vi "ODMR (with vol values).vi"() -> ()   [LabVIEW 2025]
uses:
  <vilib>/DAQmx/write.llb/DAQmx Write (Analog DBL 1Chan 1Samp).vi
  <vilib>/DAQmx/read.llb/DAQmx Read (Counter DBL 1Chan 1Samp).vi
  <vilib>/DAQmx/write.llb/DAQmx Write (Analog 1D DBL NChan 1Samp).vi
  <vilib>/DAQmx/create/channels.llb/DAQmx Create Channel (CI-Count Edges).vi
  <vilib>/DAQmx/create/channels.llb/DAQmx Create Channel (AO-Voltage-Basic).vi
  <vilib>/DAQmx/miscellaneous.llb/DAQmx Fill In Error Info.vi
  <vilib>/Utility/file.llb/Write Delimited Spreadsheet (DBL).vi
panel:
  in  "file path (dialog if empty)":path
  in  "MW stabalisation (ms)":u32
  out "interations":i32
  in  "Vx":dbl
  in  "Vy":dbl
  in  "End frequency (Ghz)":dbl
  in  "start frequency (Ghz)":dbl
  in  "Step size (Mhz)":dbl
  in  "Dwell time (ms)":u32=30
  out "XY Graph":cluster{"Y":dbl[], "Y":dbl[]}[](graph)
  out "appended array":dbl[](array[numeric])
  in  "VISA resource name":refnum<visa-resource-name>
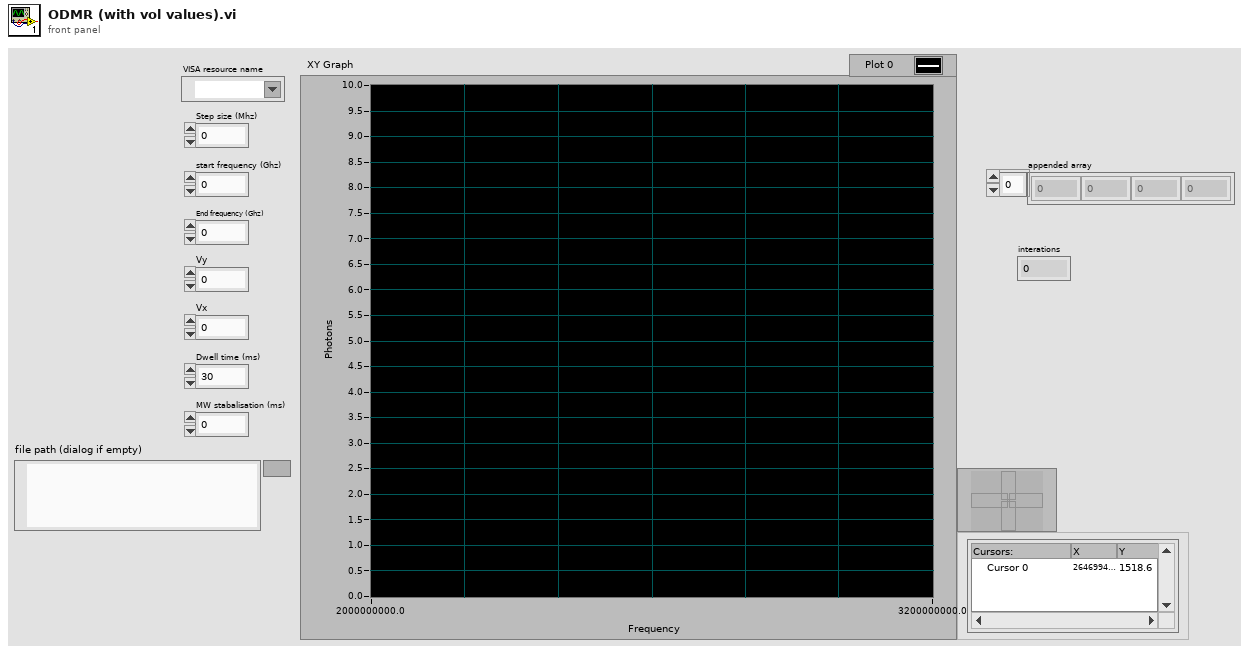
[diagram p1: front panel]
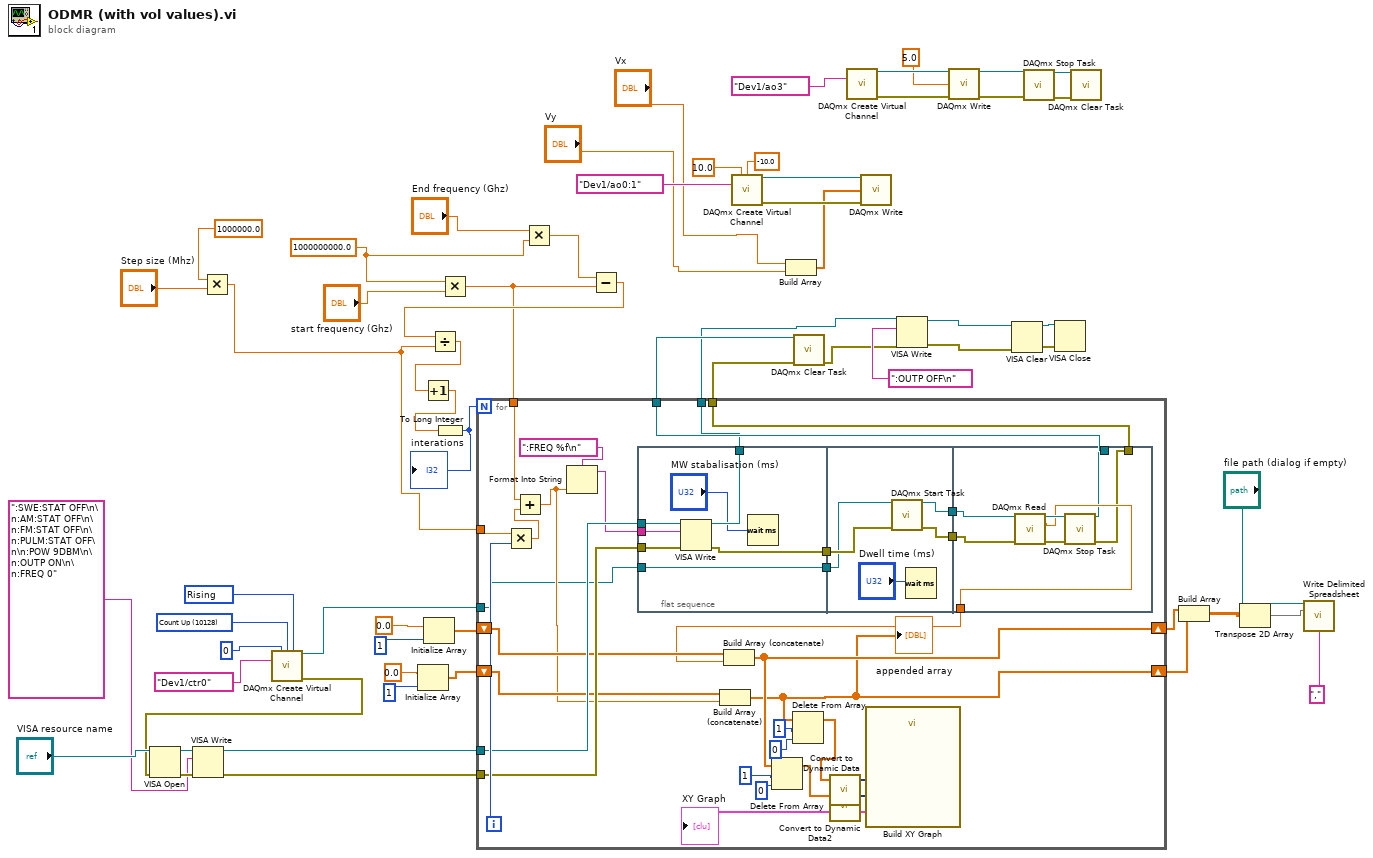
[diagram p0: block diagram]
diagram:
  w48 = 1000000000.0 ("x")
  w57 = 10128 items=["Count Up"=10128, "Count Down"=10124, "Externally Controlled"=10326] ("count direction")
  w58 = 10280 items=["Rising"=10280, "Falling"=10171] ("edge")
  n1 = Multiply(x=1000000.0, y="Step size (Mhz)") -> (x*y=w44:dbl)
  n2 = call-poly <vilib>:"DAQmx Create Virtual Channel.vi"("initial count"=u32 0, "count direction"=w57, "edge"=w58, "counter"=tag "Dev1/ctr0") -> ("task out"=w20:refnum<k21>, "error out"=w9:errorcluster)  [unwired: 10 in]
  n3 = VISA Open(error in (no error)=w9, VISA resource name="VISA resource name") -> (VISA resource name=w54:refnum<visa-resource-name>, error out=w52:errorcluster)  [unwired: 3 in]
  n4 = VISA Write(VISA resource name=w54, write buffer=":SWE:STAT OFF\n\n:AM:STAT OFF\n\n:FM:STAT OFF\n\n:PULM:STAT OFF\n\n:POW 9DBM\n\n:OUTP ON\n\n:FREQ 0", error in (no error)=w52) -> (VISA resource name out=w42:refnum<visa-resource-name>, error out=w41:errorcluster)  [unwired: 1 out]
  n5 = Initialize Array(0.0 ("element"), 1 ("dimension size")) -> (w35:dbl[])
  n6 = Initialize Array(0.0 ("element"), 1 ("dimension size")) -> (w40:dbl[])
  n7 = Multiply(x=w48, y="start frequency (Ghz)") -> (x*y=w43:dbl)
  n8 = Multiply(x="End frequency (Ghz)", y=w48) -> (x*y=w46:dbl)
  n9 = Subtract(x=w46, y=w43) -> (x-y=w45:dbl)
  n10 = Divide(x=w45, y=w44) -> (x/y=w21:dbl)
  n11 = Increment(x=w21) -> (x+1=w17:dbl)
  n12 = To Long Integer(number=w17) -> (32bit integer=w16:i32)
  "interations" <- w16
  n13 = for {
    N: w16 -> [_]
    tunnel: w44 -> [w90]
    tunnel: w43 -> [w89]
    tunnel: w42 -> [w88]
    tunnel: w41 -> [w86]
    tunnel: w20 -> [w62]
    shift-right: [w77] -> w11
    shift-left: w40 -> [w85]
    shift-right: [w74] -> w10
    shift-left: w35 -> [w84]
    tunnel: [w64] -> w34
    tunnel: [w78] -> w33
    tunnel: [w69] -> w23
    i -> [w91]
    n14 = Multiply(x=w90, y=w91) -> (x*y=w92:dbl)
    n15 = Add(x=w89, y=w92) -> (x+y=w83:dbl)
    n16 = Format Into String(format string=":FREQ %f\n" ("initial string"), w83) -> (resulting string=w87:string)  [unwired: 2 in, 1 out]
    n17 = flat-sequence {
      tunnel: w88 -> [w99]
      tunnel: w87 -> [w98]
      tunnel: w86 -> [w97]
      tunnel: [w96] -> w67
      tunnel: [w95] -> w69
      tunnel: [w94] -> w63
      tunnel: w62 -> [w94]
      tunnel: w67 -> [w104]
      tunnel: [w103] -> w66
      tunnel: [w102] -> w65
      tunnel: w63 -> [w100]
      tunnel: [w109] -> w82
      tunnel: [w108] -> w64
      tunnel: [w107] -> w78
      tunnel: w66 -> [w106]
      tunnel: w65 -> [w105]
      frame #0 {
        n18 = VISA Write(VISA resource name=w99, write buffer=w98, error in (no error)=w97) -> (VISA resource name out=w95:refnum<visa-resource-name>, error out=w96:errorcluster)  [unwired: 1 out]
        n19 = Wait (ms)(milliseconds to wait="MW stabalisation (ms)") -> ()  [unwired: 1 out]
      }
      frame #1 {
        n20 = call <vilib>:"DAQmx Start Task.vi"("task/channels in"=w100, "error in"=w104) -> ("task out"=w103:refnum<k21>, "error out"=w102:errorcluster)  [unwired: 12 in]
        n21 = Wait (ms)(milliseconds to wait="Dwell time (ms)") -> ()  [unwired: 1 out]
      }
      frame #2 {
        n22 = call-poly <vilib>:"DAQmx Read.vi"("task/channels in"=w106, "error in"=w105) -> ("task out"=w110:refnum<k21>, "data"=w109:dbl, "error out"=w111:errorcluster)  [unwired: 11 in]
        n23 = call <vilib>:"DAQmx Stop Task.vi"("task/channels in"=w110, "error in"=w111) -> ("task out"=w107:refnum<k21>, "error out"=w108:errorcluster)  [unwired: 12 in]
      }
    }
    n24 = Build Array (concatenate)(w84, w83) -> (w74:dbl[])
    "appended array" <- w74
    n25 = Build Array (concatenate)(w85, w82) -> (w77:dbl[])
    n26 = Delete From Array(array=w77, length=1, index=0) -> (array with subset deleted=w71:dbl[])  [unwired: 1 out]
    n27 = Delete From Array(array=w74, length=1, index=0) -> (array with subset deleted=w70:dbl[])  [unwired: 1 out]
    n28 = call "Convert to Dynamic Data"("Array"=w70) -> ("Dynamic Data Type"=w80:dynamicdata)  [unwired: 3 in]
    n29 = call "Convert to Dynamic Data2"("Array"=w71) -> ("Dynamic Data Type"=w79:dynamicdata)  [unwired: 3 in]
    n30 = call "Build XY Graph"("Y Input"=w79, "X Input"=w80) -> ("XY Graph"=→"XY Graph":cluster{"X":dbl[], "Y":dbl[]}[])  [unwired: 8 in, 1 out]
  }
  n31 = call-poly <vilib>:"DAQmx Create Virtual Channel.vi"("maximum value"=10.0, "minimum value"=-10.0, "physical channels"=tag "Dev1/ao0:1") -> ("task out"=w61:refnum<k21>, "error out"=w53:errorcluster)  [unwired: 11 in]
  n32 = Build Array("Vx", "Vy") -> (w32:dbl[])
  n33 = call <vilib>:"DAQmx Clear Task.vi"("task in"=w33, "error in"=w34) -> ("error out"=w22:errorcluster)  [unwired: 13 in]
  n34 = call-poly <vilib>:"DAQmx Create Virtual Channel.vi"("physical channels"=tag "Dev1/ao3") -> ("task out"=w6:refnum<k21>, "error out"=w7:errorcluster)  [unwired: 13 in]
  n35 = call-poly <vilib>:"DAQmx Write.vi"("task/channels in"=w61, "data"=w32, "error in"=w53) -> ()  [unwired: 10 in, 3 out]
  n36 = VISA Write(VISA resource name=w23, write buffer=":OUTP OFF\n", error in (no error)=w22) -> (VISA resource name out=w25:refnum<visa-resource-name>, error out=w26:errorcluster)  [unwired: 1 out]
  n37 = call-poly <vilib>:"DAQmx Write.vi"("task/channels in"=w6, "data"=5.0, "error in"=w7) -> ("task out"=w2:refnum<k21>, "error out"=w4:errorcluster)  [unwired: 10 in, 1 out]
  n38 = VISA Clear(VISA resource name=w25, error in (no error)=w26) -> (VISA resource name out=w28:refnum<visa-resource-name>, error out=w27:errorcluster)
  n39 = call <vilib>:"DAQmx Stop Task.vi"("task/channels in"=w2, "error in"=w4) -> ("task out"=w1:refnum<k21>, "error out"=w3:errorcluster)  [unwired: 12 in]
  n40 = VISA Close(VISA resource name=w28, error in (no error)=w27) -> ()  [unwired: 1 out]
  n41 = call <vilib>:"DAQmx Clear Task.vi"("task in"=w1, "error in"=w3) -> ()  [unwired: 13 in, 1 out]
  n42 = Build Array(w11, w10) -> (w14:dbl[][])
  n43 = Transpose 2D Array(2D array=w14) -> (transposed array=w13:dbl[][])
  n44 = call-poly <vilib>:"Write Delimited Spreadsheet.vi"("file path (dialog if empty)"="file path (dialog if empty)", "2D data"=w13, "delimiter (\\t)"="," ("delimiter (\\t)")) -> ()  [unwired: 11 in, 2 out]
